vi "Send Configure Interpolation [I].vi"(7 "Message Priority (Normal)":T1=enum."Normal", 8 "error in (no error)":errorcluster, 10 "interpolation":i32(ring)=1 items=["No Interpolation"=1, "sin(x)/x"=2, "Linear Interpolation"=3], 11 "Message Enqueuer":refnum<class "Message Enqueuer.lvclass">) -> (0 "error out":errorcluster, 3 "Message Enqueuer out":refnum<class "Message Enqueuer.lvclass">)   [LabVIEW 2016, in "CS++Scope.lvlib" / "Configure Interpolation [I] Msg.lvclass"]
doc: "Sends the <B>CS++Scope.lvlib:Configure Interpolation [I] Msg.lvclass</B> message.\n\n<B>CS++Scope.lvlib:CS++Scope.lvclass:Configure Interpolation [I].vi</B> Description:\n\nThis VI configures the interpolation method the oscilloscope uses when it cannot sample a voltage for a point in the waveform record. \n\nNotes:\n\n(1) This VI is part of the miscellaneous [*] extension group."
uses:
  Configure Interpolation [I] Msg.lvclass
  <vilib>/ActorFramework/Message Enqueuer/Message Enqueuer.lvclass
  <vilib>/ActorFramework/Message Enqueuer/Message Priority.ctl
  C:/Program Files (x86)/National Instruments/LabVIEW 2016/vi.lib/ActorFramework/Message/Message.lvclass
  Configure Interpolation [I] Msg.lvclass/Configure Interpolation [I] Msg.ctl
  <vilib>/ActorFramework/Message Enqueuer/Message Enqueuer.lvclass/Message Enqueuer.ctl
  <vilib>/ActorFramework/Message Priority Queue/Priority Enqueue.vi
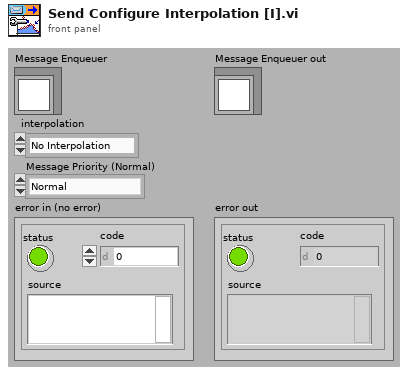
[diagram p1: front panel]
types:
  T1 = typedef "Actor Framework.lvlib/Message Enqueuer.lvclass/Message Priority.ctl" = enum16{"Low", "Normal", "High"}
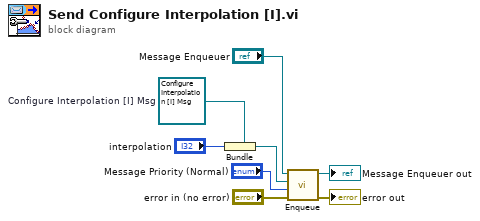
[diagram p0: block diagram]
diagram:
  w2 = refnum<class "Configure Interpolation [I] Msg.lvclass"> refnum  # Configure Interpolation [I] Msg
  n1 = Bundle(cluster=w2, "interpolation") -> (w5:refnum<class "Configure Interpolation [I] Msg.lvclass">)
  n2 = call <vilib>:"Enqueue.vi"("error in (no error)"="error in (no error)", "Message Priority (Normal)"="Message Priority (Normal)", "Message"=w5, "Message Enqueuer in"="Message Enqueuer") -> ("error out"=→"error out":errorcluster, "Message Enqueuer out"=→"Message Enqueuer out":refnum<class "Message Enqueuer.lvclass">)  [unwired: 6 in]
